vi "6133.vi"(0 "6133队列":refnum<queue>, 2 "率":dbl=1600000.0 format="%#_8g", 3 "采样数":i32=1600000, 4 "timeout (s)":dbl=10.0 caption="超时(s)" format="%0.2f", 5 "error in":errorcluster caption="错误输入", 7 "stop (F)":bool caption="停止(F)", 10 "设备名":tag="PXI1Slot3") -> (14 "task out":refnum<k21> caption="任务输出", 17 "data":sgl[][](array[numeric]) caption="数据" format="%0.2f", 18 "stopped":bool caption="已停止", 19 "error out":errorcluster caption="错误输出")   [LabVIEW 2014]
doc: "通过NI-DAQmx创建、编辑和运行任务。关于NI-DAQmx支持设备的完整列表，见NI-DAQ自述文件。\n\n在程序框图上放置DAQ助手Express VI，可通过DAQ助手新建任务。创建任务后，双击DAQ助手Express VI可编辑该任务。如需连续进行测量或信号生成，可将DAQ助手Express VI置于While循环内。"
uses:
  <vilib>/DAQmx/read.llb/DAQmx Read.vi
  <vilib>/DAQmx/read.llb/DAQmx Read (Analog 2D DBL NChan NSamp).vi
  <vilib>/DAQmx/miscellaneous.llb/DAQmx Fill In Error Info.vi
  <vilib>/DAQmx/configure/timing.llb/DAQmx Timing (Sample Clock).vi
  <vilib>/DAQmx/create/channels.llb/DAQmx Create Channel (AI-Voltage-Basic).vi
  <vilib>/DAQmx/create/channels.llb/DAQmx Create Channel (TEDS-AI-Voltage-Basic).vi
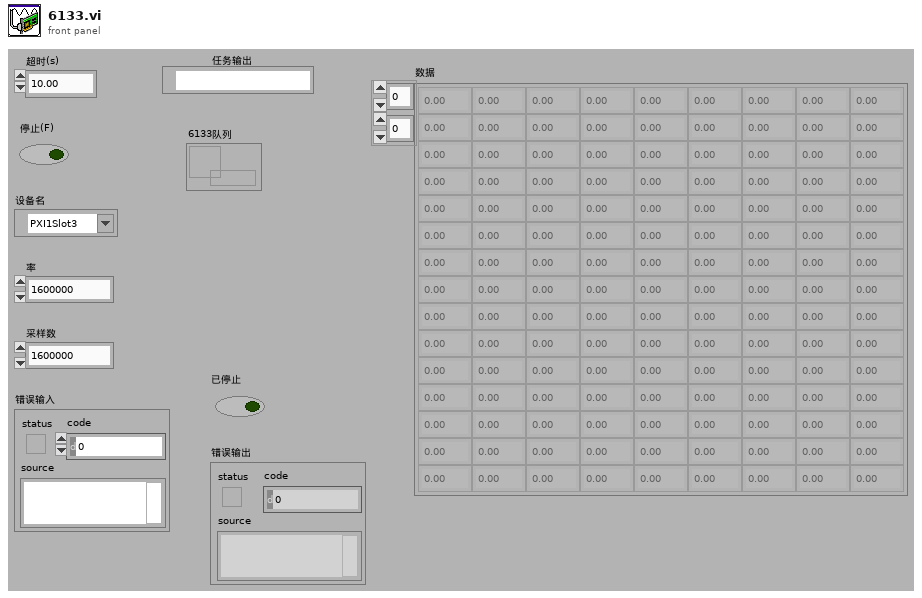
[diagram p1: front panel]
types:
  T1 = cluster{string, "seconds since 1Jan1904":timestamp, "data":dbl[][]}
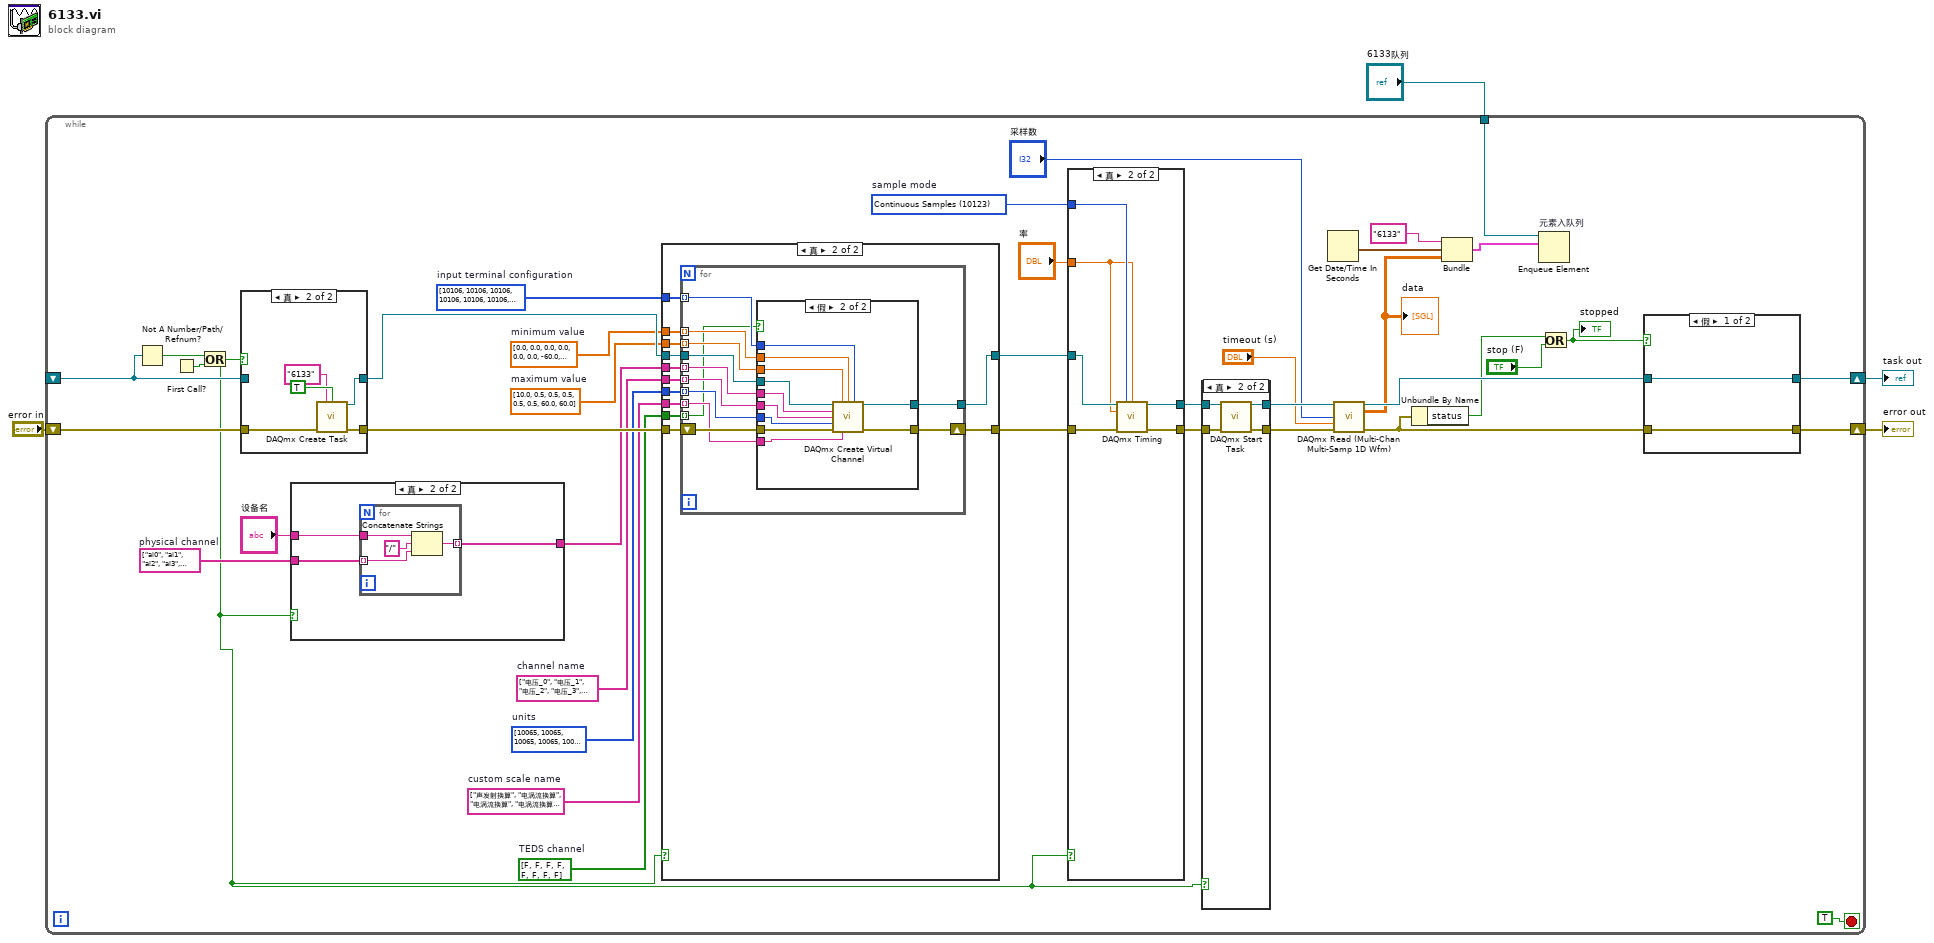
[diagram p0: block diagram]
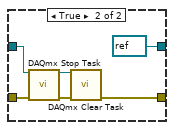
[diagram p2: hidden frame]
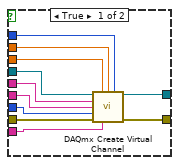
[diagram p6: hidden frame]
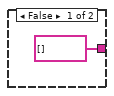
[diagram p7: hidden frame]
diagram:
  n1 = while {
    shift-right: [w17] -> w2
    shift-left: _ -> [w41]
    shift-right: [w15] -> w3
    shift-left: "error in" -> [w42]
    tunnel: "6133队列" -> [w9]
    stop <- TRUE stop-if-true
    w25 = 10123 items=["Finite Samples"=10178, "Continuous Samples"=10123, "Hardware Timed Single Point"=12522]  # sample mode
    w28 = bool[] [FALSE, FALSE, FALSE, FALSE, FALSE, FALSE, FALSE, FALSE]  # TEDS channel
    w29 = string[] ["声发射换算", "电涡流换算", "电涡流换算", "电涡流换算", "电涡流换算", "电涡流换算", "加速度换算", "加速度换算"]  # custom scale name
    w30 = i32[] [10065, 10065, 10065, 10065, 10065, 10065, 10065, 10065] items=["Volts"=10348, "From TEDS"=12516, "From Custom Scale"=10065]  # units
    w31 = string[] ["电压_0", "电压_1", "电压_2", "电压_3", "电压_4", "电压_5", "电压_6", "电压_7"]  # channel name
    w33 = dbl[] [10.0, 0.5, 0.5, 0.5, 0.5, 0.5, 60.0, 60.0]  # maximum value
    w34 = dbl[] [0.0, 0.0, 0.0, 0.0, 0.0, 0.0, -60.0, -60.0]  # minimum value
    w35 = i32[] [10106, 10106, 10106, 10106, 10106, 10106, 10106, 10106] items=["default"=-1, "RSE"=10083, "NRSE"=10078, "Differential"=10106, "Pseudodifferential"=12529]  # input terminal configuration
    w38 = string[] ["ai0", "ai1", "ai2", "ai3", "ai4", "ai5", "ai6", "ai7"]  # physical channel
    n2 = Not A Number/Path/Refnum?(number/path/refnum=w41) -> (NaN/Path/Refnum?=w40:bool)
    n3 = First Call?() -> (First Call?: T/F=w43:bool)
    n4 = Or(x=w40, y=w43) -> (x .or. y?=w24:bool)
    n5 = case "条件结构" shown="真" w24 {
      tunnel: [w124 w129] -> w37
      tunnel: w41 -> [w124 _]
      tunnel: [w123 w128] -> w36
      tunnel: w42 -> [w123 w126]
      frame False {
      }
      frame True {
        n6 = call <vilib>:"DAQmx Create Task.vi"("new task name"="6133", "auto cleanup"=TRUE, "error in"=w126) -> ("task out"=w129:refnum<k21>, "error out"=w128:errorcluster)  [unwired: 11 in]
      }
    }
    n7 = case "条件结构" shown="真" w24 {
      tunnel: [string[] [] w118] -> w32
      tunnel: "设备名" -> [_ w117]
      tunnel: w38 -> [_ w116]
      frame False {
      }
      frame True {
        n8 = for "For循环" {
          tunnel: [w122] -> w118 mode=indexing
          tunnel: w117 -> [w121]
          tunnel: w116 -> [w119] mode=indexing
          n9 = Concatenate Strings(w121, "/" ("string"), w119) -> (w122:string)
        }
      }
    }
    n10 = case "条件结构" shown="真" w24 {
      tunnel: [w68 w78] -> w27
      tunnel: w37 -> [w68 w80]
      tunnel: [w67 w77] -> w26
      tunnel: w36 -> [w67 w79]
      tunnel: w35 -> [_ w76]
      tunnel: w34 -> [_ w75]
      tunnel: w33 -> [_ w74]
      tunnel: w32 -> [_ w73]
      tunnel: w31 -> [_ w72]
      tunnel: w30 -> [_ w71]
      tunnel: w29 -> [_ w70]
      tunnel: w28 -> [_ w69]
      frame False {
      }
      frame True {
        n11 = for "For循环" {
          tunnel: w80 -> [w92]
          tunnel: [w90] -> w78
          tunnel: w76 -> [w88] mode=indexing
          tunnel: w75 -> [w87] mode=indexing
          tunnel: w74 -> [w86] mode=indexing
          tunnel: w73 -> [w85] mode=indexing
          tunnel: w72 -> [w84] mode=indexing
          tunnel: w71 -> [w83] mode=indexing
          tunnel: w70 -> [w82] mode=indexing
          shift-right: [w89] -> w77
          shift-left: w79 -> [w91]
          tunnel: w69 -> [w81] mode=indexing
          n12 = case "条件结构" shown="假" w81 {
            tunnel: w92 -> [w103 w114]
            tunnel: w91 -> [w102 w113]
            tunnel: [w101 w112] -> w90
            tunnel: [w100 w111] -> w89
            tunnel: w88 -> [w99 w110]
            tunnel: w87 -> [w98 w109]
            tunnel: w86 -> [w97 w108]
            tunnel: w85 -> [w96 w107]
            tunnel: w84 -> [w95 w106]
            tunnel: w83 -> [w94 w105]
            tunnel: w82 -> [w93 w104]
            frame True {
              n13 = call-poly <vilib>:"DAQmx Create Virtual Channel.vi"("task in"=w103, "maximum value"=w97, "minimum value"=w98, "input terminal configuration"=w99, "physical channels"=w96, "name to assign"=w95, "units"=w94, "error in"=w102, "custom scale name"=w93) -> ("task out"=w101:refnum<k21>, "error out"=w100:errorcluster)  [unwired: 5 in]
            }
            frame False {
              n14 = call-poly <vilib>:"DAQmx Create Virtual Channel.vi"("task in"=w114, "maximum value"=w108, "minimum value"=w109, "input terminal configuration"=w110, "physical channels"=w107, "name to assign"=w106, "units"=w105, "error in"=w113, "custom scale name"=w104) -> ("task out"=w112:refnum<k21>, "error out"=w111:errorcluster)  [unwired: 5 in]
            }
          }
        }
      }
    }
    n15 = case "条件结构" shown="真" w24 {
      tunnel: [w60 w63] -> w23
      tunnel: w27 -> [w60 w65]
      tunnel: [w59 w62] -> w22
      tunnel: w26 -> [w59 w64]
      tunnel: w25 -> [_ w66]
      tunnel: "率" -> [_ w61]
      frame False {
      }
      frame True {
        n16 = call-poly <vilib>:"DAQmx Timing.vi"("task/channels in"=w65, "sample mode"=w66, "samples per channel"=w61, "rate"=w61, "error in"=w64) -> ("task out"=w63:refnum<k21>, "error out"=w62:errorcluster)  [unwired: 9 in]
      }
    }
    n17 = case "条件结构" shown="真" w24 {
      tunnel: [w54 w57] -> w21
      tunnel: w23 -> [w54 w58]
      tunnel: [w53 w55] -> w20
      tunnel: w22 -> [w53 w56]
      frame False {
      }
      frame True {
        n18 = call <vilib>:"DAQmx Start Task.vi"("task/channels in"=w58, "error in"=w56) -> ("task out"=w57:refnum<k21>, "error out"=w55:errorcluster)  [unwired: 12 in]
      }
    }
    n19 = Get Date/Time In Seconds ("获取日期/时间（秒）")() -> (seconds since 1Jan1904=w8:timestamp)
    n20 = call-poly "DAQmx Read (Multi-Chan Multi-Samp 1D Wfm).vi"("task/channels in"=w21, "number of samples per channel"="采样数", "timeout"="timeout (s)", "error in"=w20) -> ("task out"=w16:refnum<k21>, "data"=w5:dbl[][], "error out"=w14:errorcluster)  [unwired: 9 in]
    "data" <- w5
    n21 = Unbundle By Name(w14) -> ("status"=w13:bool)
    n22 = Bundle("6133", "seconds since 1Jan1904"=w8, "data"=w5) -> (w6:T1)  [unwired: 1 in]
    n23 = Enqueue Element "元素入队列"(queue=w9, element=w6) -> ()  [unwired: 2 in, 3 out]
    n24 = Or(x=w13, y="stop (F)") -> (x .or. y?=w11:bool)
    "stopped" <- w11
    n25 = case "条件结构" shown="假" w11 {
      tunnel: [w46 refnum<k21> refnum ("task in")] -> w17
      tunnel: w16 -> [w46 w52]
      tunnel: [w45 w49] -> w15
      tunnel: w14 -> [w45 w51]
      frame False {
      }
      frame True {
        n26 = call <vilib>:"DAQmx Stop Task.vi"("task/channels in"=w52, "error in"=w51) -> ("task out"=w48:refnum<k21>, "error out"=w50:errorcluster)  [unwired: 12 in]
        n27 = call <vilib>:"DAQmx Clear Task.vi"("task in"=w48, "error in"=w50) -> ("error out"=w49:errorcluster)  [unwired: 13 in]
      }
    }
  }
  "error out" <- w3
  "task out" <- w2
